vi "Update.vi"(8 "error in (no error)":errorcluster, 10 "Simulation Objects in":refnum<class "SimulationObject.lvclass">[](array[class]), 11 "DrawingSystem in":refnum<class "DrawingSystem.lvclass">) -> (0 "error out":errorcluster, 2 "Simulation Objects out":refnum<class "SimulationObject.lvclass">[](array[class]), 3 "DrawingSystem out":refnum<class "DrawingSystem.lvclass">)   [LabVIEW 2022 SP3, in "DrawingSystem.lvclass"]
uses:
  DrawingSystem.lvclass
  Objects/SimulationObject/SimulationObject.lvclass
  DrawingSystem.lvclass/DrawingSystem.ctl
  Math/Vector2/Vector2.lvclass
  Objects/Components/DrawComponent/DrawComponent.lvclass
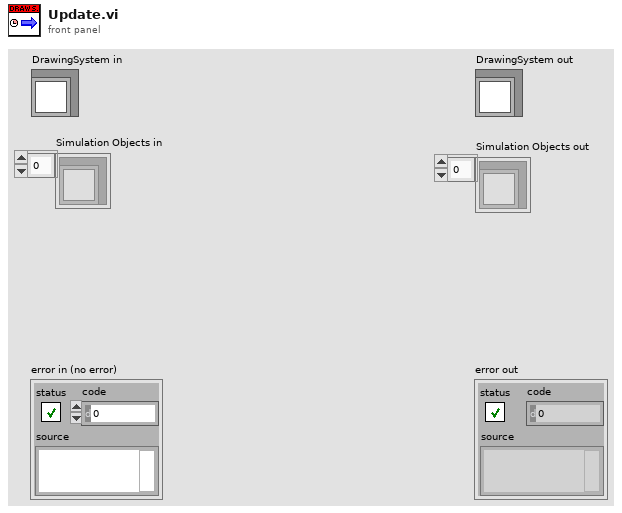
[diagram p1: front panel]
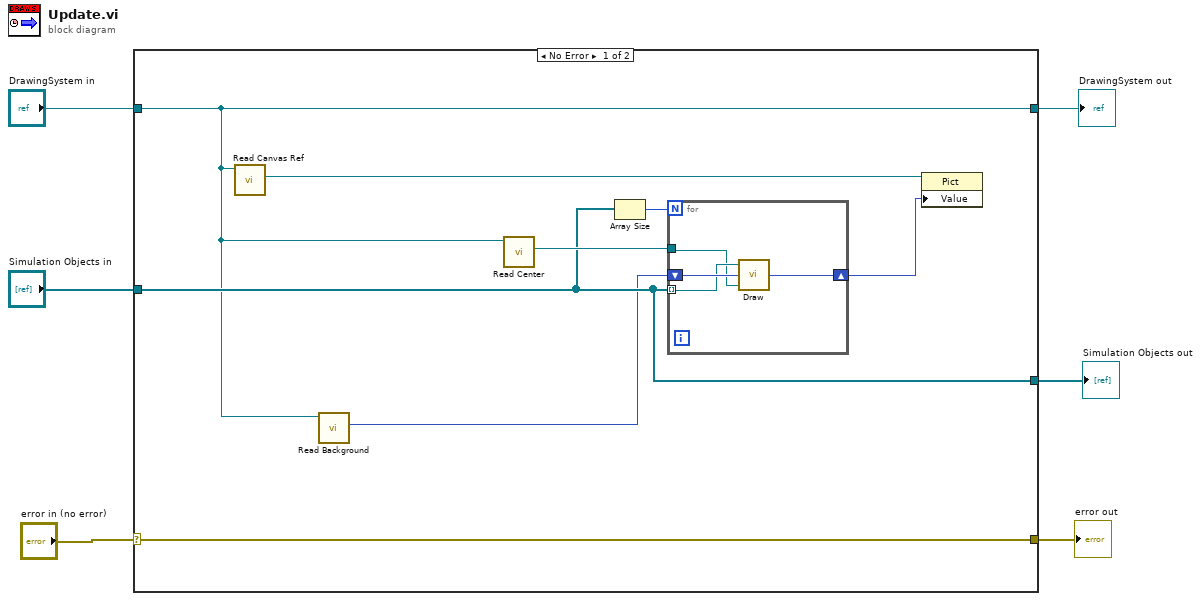
[diagram p0: block diagram]
diagram:
  n1 = case shown="No Error" "error in (no error)" {
    selector: "error in (no error)" -> [w14 w21]
    tunnel: [w14 w21] -> w5
    tunnel: [w8 w20] -> w3
    tunnel: "DrawingSystem in" -> [w8 w20]
    tunnel: "Simulation Objects in" -> [w10 w19]
    tunnel: [w10 w19] -> w1
    frame No Error {
      n2 = call "Read Canvas Ref.vi"("DrawingSystem in"=w8) -> ("Canvas Ref"=w9:refnum<vi>)  [unwired: 8 in, 2 out]
      n3 = call "Read Background.vi"("DrawingSystem in"=w8) -> ("Background"=w7:picture)  [unwired: 8 in, 2 out]
      n4 = call "Read Center.vi"("DrawingSystem in"=w8) -> ("Vector2.lvclass"=w11:refnum<class "Vector2.lvclass">)  [unwired: 8 in, 2 out]
      n5 = Array Size(array=w10) -> (size(s)=w12:i32)
      n6 = for {
        N: w12 -> [_]
        shift-right: [w18] -> w13
        shift-left: w7 -> [w17]
        tunnel: w10 -> [w16] mode=indexing
        tunnel: w11 -> [w15]
        n7 = call "Draw.vi"("Center position in"=w15, "Picture in"=w17, "Simulation Object in"=w16) -> ("Picture out"=w18:picture)
      }
      n8 = property class="Pict"(reference=w9, "Value"=w13) -> ()  [unwired: 1 in, 2 out]
    }
    frame Error {
    }
  }
  "error out" <- w5
  "DrawingSystem out" <- w3
  "Simulation Objects out" <- w1
